vi "CameraVision.vi"(8 "error in (no error)":errorcluster, 9 "Com-in":refnum<queue>, 10 "Com-out":refnum<queue>) -> (0 "error out":errorcluster)   [LabVIEW 2013, in "CameraVision.lvlib"]
doc: "This vi is the main component of the CameraVision software.\n\nThe software is made for the acquisition, processing and storage of images. Specifically using one or two CMOS cameras and a SiliconSoftware framegrabber. The cameras can be any type compatible with the framegrabber, though the software is only tested with PhotonFocus CMOS-cameras of the MV-D1312-240-CL model. In this case a separate software called 'PFRemote', provided by PhotonFocus, is necessary for changing camera parameters.\n\nThe main program controls are on the top of the window. User-configurable settings are grouped per category on the left panel. All outputs are displayed at the right side of the window. Different display configurations can be chosen using the tabs."
uses:
  CameraVision.lvlib
  Sources/UI/Settings-source.ctl
  Sources/UI/Camera-selector.ctl
  Sources/UI/Image-selector.ctl
  Sources/Main/Configuration/Configuration-parameters-gui.ctl
  Sources/Main/Storage/Storage-parameters-gui.ctl
  Sources/Main/Storage/Storage-types.ctl
  Sources/Main/Acquisition/Acquisition-parameters-gui.ctl
  Sources/Main/Acquisition/Trigger-modes.ctl
  Sources/Main/Acquisition/Exposure-modes.ctl
  Sources/Main/Analysis/Characteristics-cluster.ctl
  Sources/Main/Correction/Correction-parameters-gui.ctl
  Sources/Main/Correction/Smoothing.ctl
  Sources/Main/Correction/Background-correction.ctl
  Sources/Main/Analysis/Analysis-parameters-gui.ctl
  Sources/Main/Temperature/Temperature-parameters-gui.ctl
  Sources/Main/Mapping/Mapping-parameters-gui.ctl
  Sources/Main/Mapping/Mapping-characteristic.ctl
  Sources/Main/Temperature/Temperature-characteristics.ctl
  SA-SLMAPI/Sources/Message.lvclass
  Sources/UI/Status-overview.ctl
  Sources/UI/Module-states.ctl
  Sources/Main/Filter/Filter-parameters-gui.ctl
  Sources/Main/Filter/Filter-settings.ctl
  Sources/Main/Filter/Filter-characteristic.ctl
  Sources/Main/Filter/Filter-apply.ctl
  Sources/Main/Main-actions.ctl
  Sources/Main/Application-states.ctl
  Sources/Main/CV-Main.lvclass
  Sources/UI/CV-UI.lvclass
  Sources/Main/Configuration/CV-Configuration.lvclass
  Sources/Main/Storage/CV-Storage.lvclass
  Sources/Main/Acquisition/CV-Acquisition.lvclass
  Sources/Main/Analysis/CV-Analysis.lvclass
  Sources/Main/Correction/CV-Correction.lvclass
  Sources/Main/Temperature/CV-Temperature.lvclass
  Sources/Main/Mapping/CV-Mapping.lvclass
  Sources/Main/Filter/CV-Filter.lvclass
panel:
  in  "Start acquisition":bool
  in  "Manual trigger":bool
  in  "Camera selector":T1 caption="Display camera"
  in  "Image type selector":T2 caption="Display image"
  in  "Batch browser":i32(slide) caption="Browse batch" min=-29 max=0 step=1
  in  "Image refresh":bool
  in  "Import images":bool
  in  "Save settings":bool
  in  "Load settings":bool
  in  "Settings type":T3
  in  "Stop acquisition":bool
  in  "Activate":bool
  in  "Show info":bool
  in  "Parameter tabs":T4(tab) caption="Parameters"
  in  "Configuration params":T5={"Number of cameras"=1, "Camera 1 port"=enum."A", "ROI width"=1248, "ROI height"=1082, "Reset ROI"=FALSE, "Width scale"=0.05, "Height scale"=0.05, "Center Y cam. 1"=541, "Center X cam. 1"=624, "Center Y cam. 2"=541, "Center X cam. 2"=624} {"Center X cam. 2" min=4 max=1244 step=8; "Center Y cam. 2" min=1 max=1082 step=1; "Center X cam. 1" min=4 max=1244 step=8; "Center Y cam. 1" min=1 max=1082 step=1; "Height scale" min=0.001 step=0.001 format="%.3f"; "Width scale" min=0.001 step=0.001 format="%.3f"; "Number of cameras" min=1 max=2 step=1; "ROI width" min=8 max=1248 step=8; "ROI height" min=1 max=1082 step=1}
  in  "Acquisition params":T6={"Acquisition mode"=enum."Continuous", "Batch size"=0, "Image buffer size"=0, "Trigger mode"=enum."Camera timed (not sync.)", "Duration HH"=1.0, "Acquisition start"=enum."Immediate", "Duration SS"=0.0, "Duration MM"=0.0, "Start time"=timestamp(0 s since 1904-01-01), "Max. frame rate"=5.0, "Exposure time cam. 1"=1.0, "Exposure time cam. 2"=1.0, "Exposure mode"=enum."Linear", "Value 1"=17.0, "Value 2"=14.0, "Time 1"=1000.0, "Time 2"=1000.0} {"Exposure time cam. 2" min=0.01 step=0.01 format="%#.2g"; "Exposure time cam. 1" min=0.01 step=0.01 format="%#.2g"; "Max. frame rate" min=0.0001 max=1000000.0 format="%#.4g"; "Start time" format="%<%X\n%x>T"; "Duration MM" min=0 max=59 step=1 format="%02.0f"; "Duration SS" min=0 max=59 step=1 format="%02.0f"; "Duration HH" min=0 step=1 format="%02.0f"; "Image buffer size" min=1 max=10000 step=1 format="%#.0f"; "Batch size" min=1 max=50000 step=1}
  in  "Processing selector":u32(ring) items=["Correction", "Analysis", "Temperature", "Mapping"]
  in  "Processing tabs":T9(tab)
  in  "Correction params":T10={"Background correction"=FALSE, "Hot-pixel correction"=FALSE, "Black image cam. 1"=path "C:/CameraVision/Black images/Black-CameraA-Full.bmp", "Black image cam. 2"=path "C:/CameraVision/Black images/Black-CameraB-Full.bmp", "Y-shift"=0, "X-shift"=0, "Correlation algorithm"=enum."Fixed shift", "Noise treshold"=25.0, "Smoothing algorithm"=enum."Noise tresholding", "2nd image correlation"=FALSE, "Image smoothing"=FALSE, "Background correction method"=enum."Hardware"} {"Noise treshold" min=0 max=255 step=1}
  in  "Analysis params":T13={"Binarization treshold"=150.0, "Image characteristics"=FALSE, "Melt-pool characteristics"=FALSE} {"Binarization treshold" min=0 max=255 step=1}
  in  "Temperature params":T14={"Temperature field"=FALSE, "Ratio correction factor"=1.0, "Temperature value"=FALSE, "Y-coord."=0.0, "X-coord."=0.0, "Averaging center"=enum."Melt-pool center", "Averaging shape"=enum."Point", "Minor axis"=0.0, "Major axis"=0.0} {"Major axis" min=0.0; "Minor axis" min=0.0; "Ratio correction factor" min=0.0 step=0.0001 format="%#.4g"}
  in  "Mapping params":T15 {"Jump speed" min=1; "Default mark speed" min=1; "Start off-set" step=0.0001}
  in  "Storage params":T17={"Base file name"="Test", "Storage directory"=path "C:/CameraVision/Results", "Save what?"={"Original"=FALSE, "Corrected"=FALSE, "Binary"=FALSE, "Temperature"=FALSE, "Characteristics"=FALSE, "Mapping"=FALSE, "TemperatureValues"=FALSE}, "Image file type"=enum."PNG", "Comments"="", "Storage mode"=enum."1 file for all layers ", "Start iteration/layer"=0}
  in  "Filter params":T19
  out "Storage buffer":dbl(slide) scale=0.0..1.0
  out "Framerate":dbl caption="Frame rate [fps]" format="%06.1f"
  out "Status overview":T23
  out "Frametime":dbl caption="Process time [ms/frame]" format="%04.0g"
  out "Process buffer":dbl(slide) scale=0.0..1.0
  out "Total disk space":dbl caption="Total [GB]" format="%05.1f"
  out "Free disk space":dbl caption="Free [GB]    /" format="%05.1f"
  out "Current image":i32 caption="Current image #" format="%06.0f"
  in  "Displays":T25(tab)=enum."Dual view"
  out "Browser":T26(plugin-control)
  out "Camera 2":T26(plugin-control)
  out "Camera 1":T26(plugin-control)
  out "Temper characteristics":T27 caption="Temperature" {"Stand. dev. temperature" format="%#.1f"; "Min. temperature" format="%#.0f"; "Max. temperature" format="%#.0f"; "Average temperature" format="%#.0f"}
  out "Characteristics":T28 caption="Image/melt-pool"
  out "Histogram":T29(graph)
  out "Information":T26(plugin-control)
  out "Camera 2 chart":dbl[][](graph) caption="Camera 2 - characteristics chart"
  out "Camera 1 chart":dbl[][](graph) caption="Camera 1 - characteristics chart"
  out "Temperature":dbl[][](graph) caption="Temperature [°C]"
  out "Map":dbl[][](graph)
  in  "Map characteristic":T16
  out "State":string caption="Status:"
  out "Action":string caption="Action:"
  # ":"
  # ":"
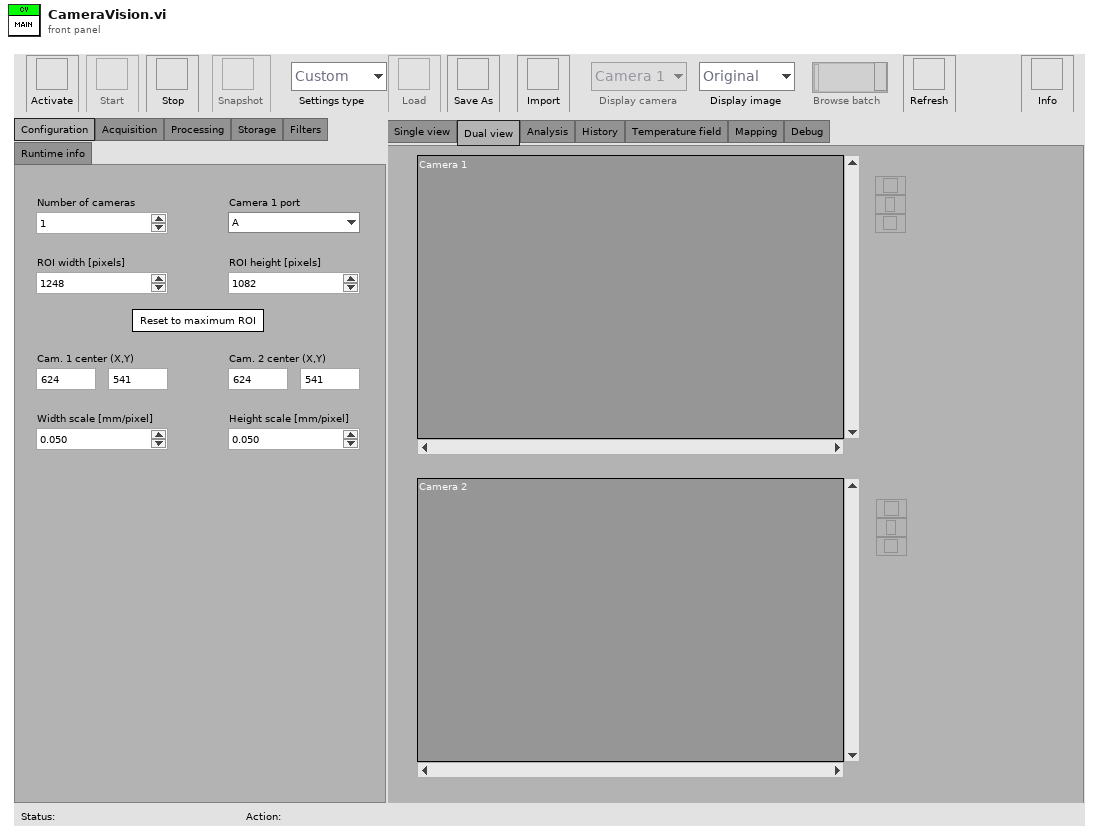
[diagram p1: front panel]
types:
  T1 = typedef "CameraVision.lvlib/CV-UI.lvclass/Camera-selector.ctl" = enum16{"Camera 1", "Camera 2"}
  T2 = typedef "CameraVision.lvlib/CV-UI.lvclass/Image-selector.ctl" = enum16{"Original", "Corrected", "Binary"}
  T3 = typedef "CameraVision.lvlib/CV-UI.lvclass/Settings-source.ctl" = enum16{"Custom", "Default", "Last used", "File"}
  T4 = enum32{"Configuration", "Acquisition", "Processing", "Storage", "Filters", "Runtime info"}
  T5 = typedef "CameraVision.lvlib/CV-Configuration.lvclass/Configuration-parameters-gui.ctl" = cluster{"Number of cameras":i32, "Camera 1 port":enum16{"A", "B"}, "ROI width":u32, "ROI height":u32, "Reset ROI":bool, "Width scale":dbl, "Height scale":dbl, "Center Y cam. 1":i32, "Center X cam. 1":i32, "Center Y cam. 2":i32, "Center X cam. 2":i32}
  T6 = typedef "CameraVision.lvlib/CV-Acquisition.lvclass/Acquisition-parameters-gui.ctl" = cluster{"Acquisition mode":enum16{"Continuous", "Continuous batch", "Single batch", "Single batch -delayed"}, "Batch size":i32, "Image buffer size":i32, "Trigger mode":T7, "Duration HH":sgl, "Acquisition start":enum16{"Immediate", "Post-phoned"}, "Duration SS":sgl, "Duration MM":sgl, "Start time":timestamp, "Max. frame rate":dbl, "Exposure time cam. 1":dbl, "Exposure time cam. 2":dbl, "Exposure mode":T8, "Value 1":dbl, "Value 2":dbl, "Time 1":dbl, "Time 2":dbl}
  T7 = typedef "CameraVision.lvlib/CV-Acquisition.lvclass/Trigger-modes.ctl" = enum16{"Camera timed (not sync.)", "Framegrabber timed (sync.)", "Software timed (sync.)", "External timing (sync.)", "Manual (sync.)", "Gated - camera (not sync.)", "Gated - grabber (sync.)", "Gated - software (sync.)", "Gated - external (sync.)"}
  T8 = typedef "CameraVision.lvlib/CV-Acquisition.lvclass/Exposure-modes.ctl" = enum16{"Linear", "LinLog"}
  T9 = enum32{"Correction", "Analysis", "Temperature", "Mapping"}
  T10 = typedef "CameraVision.lvlib/CV-Correction.lvclass/Correction-parameters-gui.ctl" = cluster{"Background correction":bool, "Hot-pixel correction":bool, "Black image cam. 1":path, "Black image cam. 2":path, "Y-shift":i32, "X-shift":i32, "Correlation algorithm":enum16{"Fixed shift", "Cross-correlation", "Cross-correlation (5steps)", "Melt-pool center"}, "Noise treshold":sgl, "Smoothing algorithm":T11, "2nd image correlation":bool, "Image smoothing":bool, "Background correction method":T12}
  T11 = typedef "CameraVision.lvlib/CV-Correction.lvclass/Smoothing.ctl" = enum16{"Noise tresholding", "NT+Median filter", "NT+Gaussian filter"}
  T12 = typedef "CameraVision.lvlib/CV-Correction.lvclass/Background-correction.ctl" = enum16{"Hardware", "Software"}
  T13 = typedef "CameraVision.lvlib/CV-Analysis.lvclass/Analysis-parameters-gui.ctl" = cluster{"Binarization treshold":sgl, "Image characteristics":bool, "Melt-pool characteristics":bool}
  T14 = typedef "CameraVision.lvlib/CV-Temperature.lvclass/Temperature-parameters-gui.ctl" = cluster{"Temperature field":bool, "Ratio correction factor":dbl, "Temperature value":bool, "Y-coord.":dbl, "X-coord.":dbl, "Averaging center":enum16{"Fixed coordinates (pixel)", "Fixed coordinates (mm)", "Melt-pool center"}, "Averaging shape":enum16{"Point", "Circle", "Ellipse"}, "Minor axis":dbl, "Major axis":dbl}
  T15 = typedef "CameraVision.lvlib/CV-Mapping.lvclass/Mapping-parameters-gui.ctl" = cluster{"Enable mapping":bool, "Automatic timing":bool, "Scan pattern file":path, "Start off-set":dbl, "Default map characteristic":T16, "Default mark speed":i32, "Jump speed":i32}
  T16 = typedef "CameraVision.lvlib/CV-Mapping.lvclass/Mapping-characteristic.ctl" = enum16{"Average intensity [0-255]", "Peak intensity [0-255]", "Melt-pool size [mm²]", "Melt-pool aspect ratio []", "Melt-pool fragments []", "Average temperature [°C]", "Max. temperature [°C]", "Min. temperature [°C]", "Std. dev. temperature [°C]"}
  T17 = typedef "CameraVision.lvlib/CV-Storage.lvclass/Storage-parameters-gui.ctl" = cluster{"Base file name":string, "Storage directory":path, "Save what?":T18, "Image file type":enum16{"JPG", "BMP", "PNG"}, "Comments":string, "Storage mode":enum16{"1 file per layer", "1 file for all layers "}, "Start iteration/layer":u16}
  T18 = typedef "CameraVision.lvlib/CV-Storage.lvclass/Storage-types.ctl" = cluster{"Original":bool, "Corrected":bool, "Binary":bool, "Temperature":bool, "Characteristics":bool, "Mapping":bool, "TemperatureValues":bool}
  T19 = typedef "CameraVision.lvlib/CV-Filter.lvclass/Filter-parameters-gui.ctl" = cluster{"Filter array":T20[], "Storage filters":T22}
  T20 = typedef "CameraVision.lvlib/CV-Filter.lvclass/Filter-settings.ctl" = cluster{"Characteristic":T21, "Monitor":bool, "Min.":dbl, "Max.":dbl, "Min. Thres.":dbl, "Min. Dur.":u16, "Report":bool}
  T21 = typedef "CameraVision.lvlib/CV-Filter.lvclass/Filter-characteristic.ctl" = enum16{"Average intensity [0-255]", "Peak intensity [0-255]", "Melt-pool size [mm²]", "Melt-pool aspect ratio []", "Melt-pool fragments []", "Melt-pool position X [pixel]", "Melt-pool position Y [pixel]", "Average temperature [°C]", "Max. temperature [°C]", "Min. temperature [°C]", "Std. dev. temperature [°C]"}
  T22 = typedef "CameraVision.lvlib/CV-Filter.lvclass/Filter-apply.ctl" = cluster{"Filter images":bool, "Filter characteristics":bool, "Filter temperature":bool}
  T23 = typedef "CameraVision.lvlib/CV-UI.lvclass/Status-overview.ctl" = cluster{"Camera hardware":T24, "Framegrabber":T24, "External timing":T24, "Image acquisition":T24, "Image processing ":T24, "Temperature":T24, "Map":T24, "Storage filter":T24, "Image storage":T24, "Charact. storage":T24, "Temperature storage":T24, "Camera hardware G":bool, "Camera hardware R":bool, "Framegrabber G":bool, "Framegrabber R":bool, "External timing G":bool, "External timing R":bool, "Image acquisition G":bool, "Image acquisition R":bool, "Image processing G":bool, "Image processing R":bool, "Temperature G":bool, "Temperature R":bool, "Map G":bool, "Map R":bool, "Storage filter G":bool, "Storage filter R":bool, "Image storage G":bool, "Image storage R":bool, "Charact storage G":bool, "Charact storage R":bool, "Temperature storage G":bool, "Temperature storage R":bool}
  T24 = typedef "CameraVision.lvlib/CV-UI.lvclass/Module-states.ctl" = enum16{"Inactive", "Active", "Data-loss", "Error", "Simulation", "Synchronizing", "Initialized", "Released"}
  T25 = enum32{"Single view", "Dual view", "Analysis", "History", "Temperature field", "Mapping", "Debug"}
  T26 = typedef "IMAQ Image.ctl" = refnum<image>
  T27 = typedef "CameraVision.lvlib/CV-Temperature.lvclass/Temperature-characteristics.ctl" = cluster{"Average temperature ":dbl, "Max. temperature":dbl, "Min. temperature":dbl, "Stand. dev. temperature":dbl, "Datapoints":dbl}
  T28 = typedef "CameraVision.lvlib/CV-Analysis.lvclass/Characteristics-cluster.ctl" = cluster{"Average intensity":dbl, "Peak intensity":dbl, "Melt-pool size":dbl, "Melt-pool aspect ratio":dbl, "Melt-pool fragments":dbl, "Centre of mass X":dbl, "Centre of mass Y":dbl, "Orientation":dbl}
  T29 = cluster{"Starting Value":sgl, "Incremental Value":sgl, "Histogram":u32[]}
  T30 = typedef "CameraVision.lvlib/CV-Main.lvclass/Main-actions.ctl" = enum16{"Idle", "Initialize", "Load defaults", "Update settings", "Check settings", "Save settings", "Save settings with dialog", "Load settings", "Load data", "Activate", "Start", "Wait for start signal", "Acquire & process", "Iterate", "Stop", "Refresh display", "Refresh status", "View camera settings", "View grabber settings", "Exit"}
  T31 = typedef "CameraVision.lvlib/CV-Main.lvclass/Application-states.ctl" = enum16{"Idle", "Initialized", "Configured", "Activated", "Started", "Stopped", "Reset", "Error", "Exited"}
  T32 = enum16{"Continuous", "Continuous batch", "Single batch", "Single batch -delayed"}
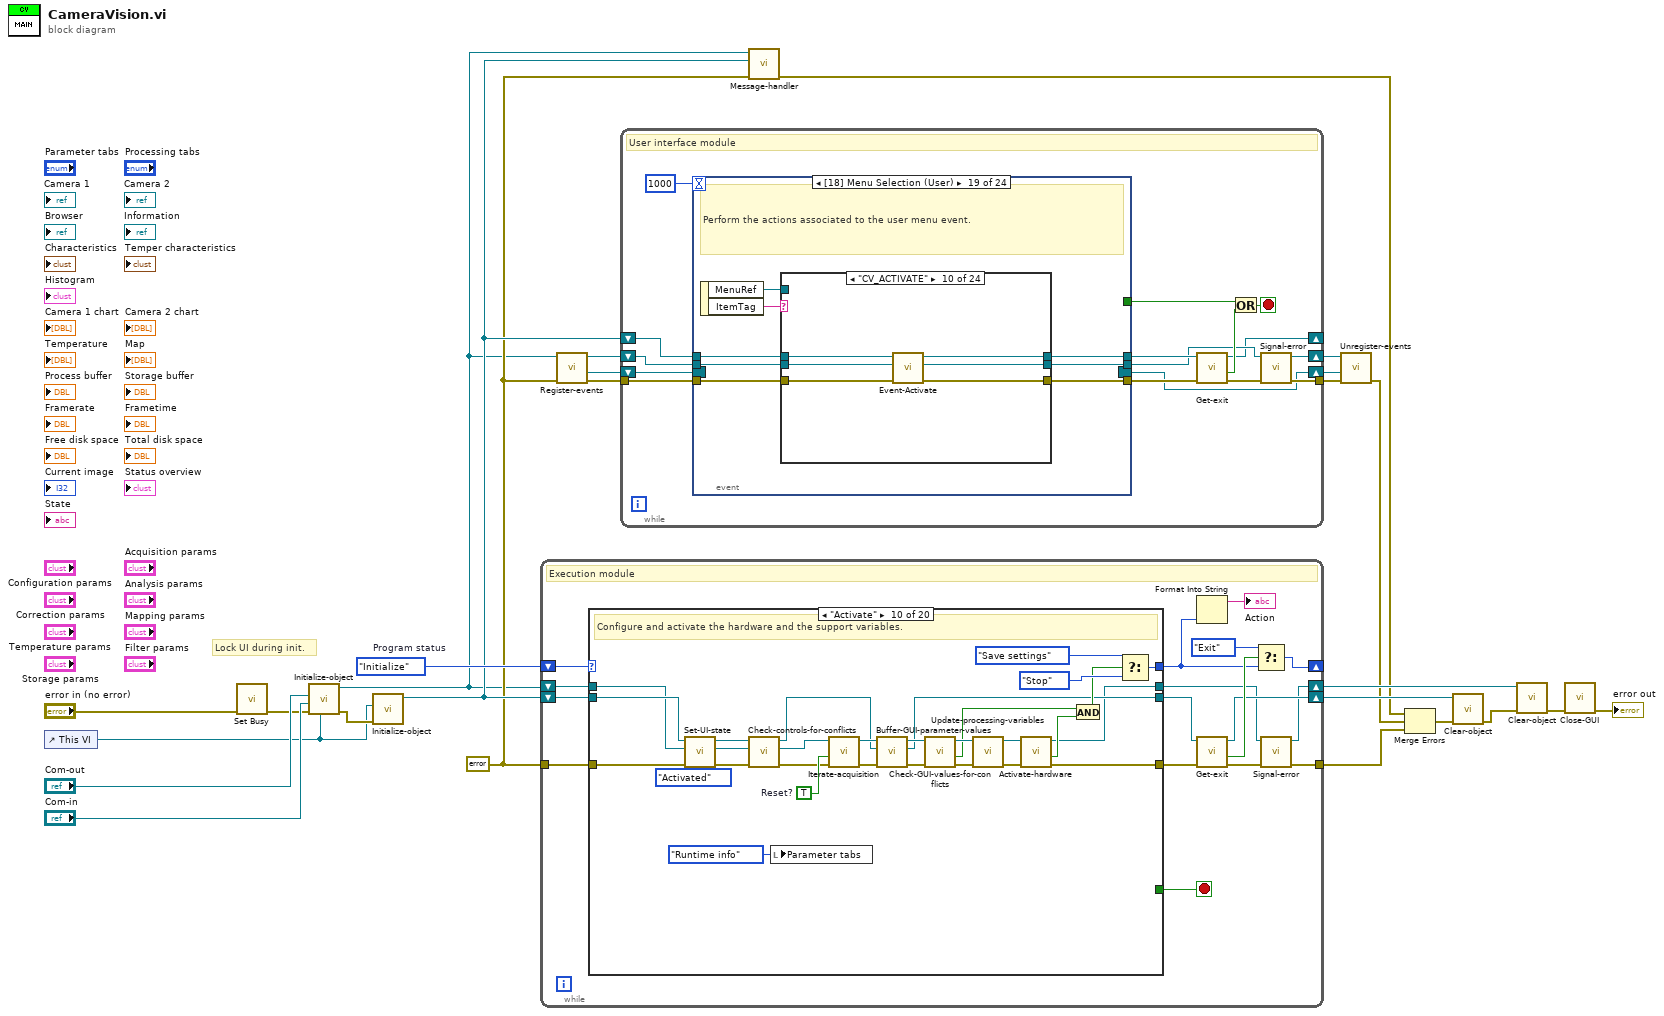
[diagram p0: block diagram]
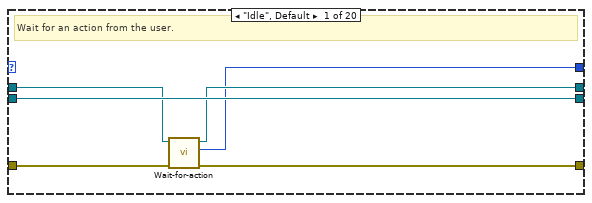
[diagram p2: hidden frame]
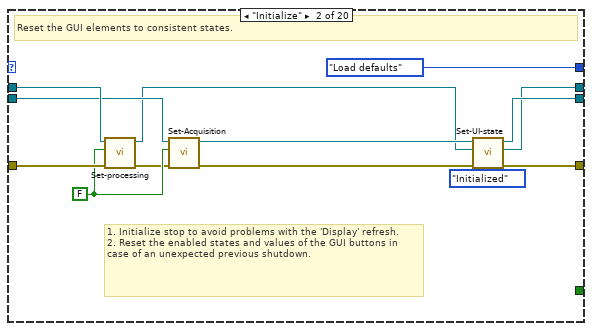
[diagram p3: hidden frame]
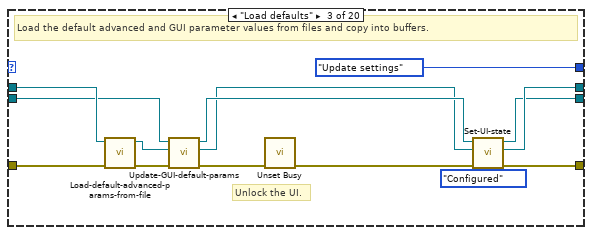
[diagram p4: hidden frame]
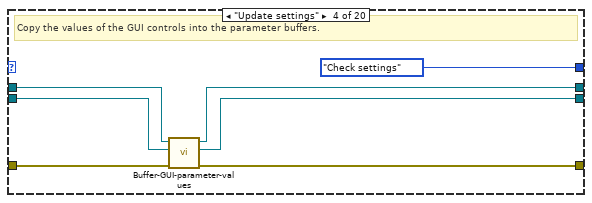
[diagram p5: hidden frame]
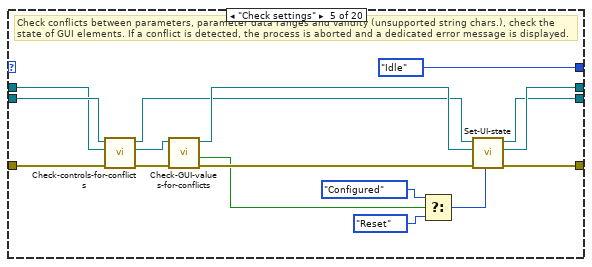
[diagram p6: hidden frame]
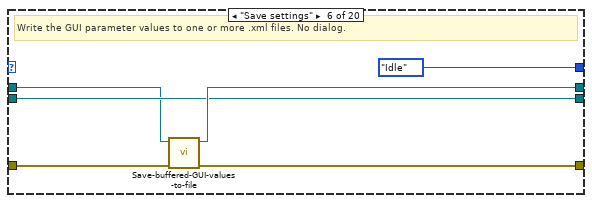
[diagram p7: hidden frame]
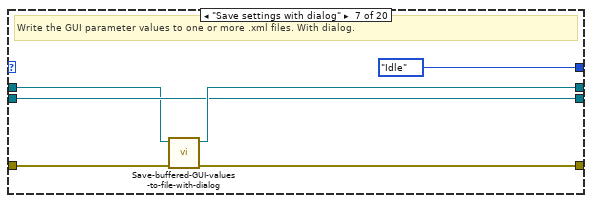
[diagram p8: hidden frame]
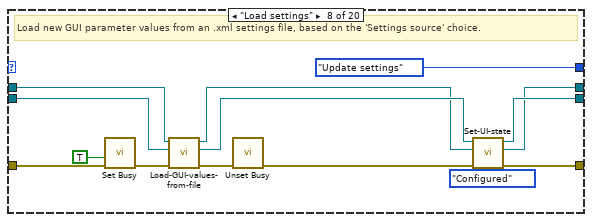
[diagram p9: hidden frame]
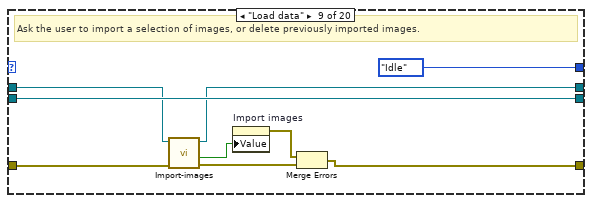
[diagram p10: hidden frame]
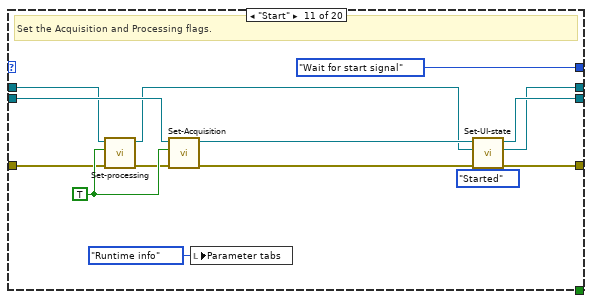
[diagram p11: hidden frame]
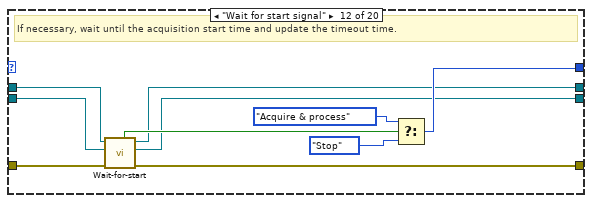
[diagram p12: hidden frame]
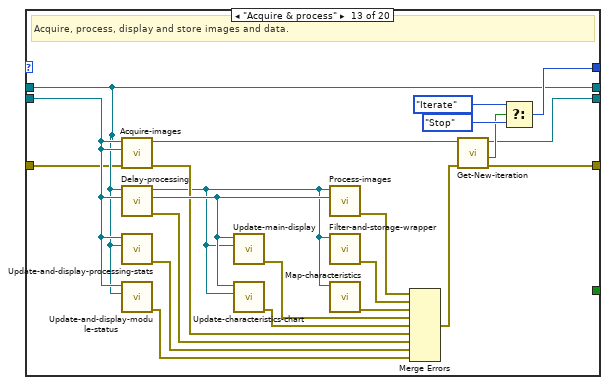
[diagram p13: hidden frame]
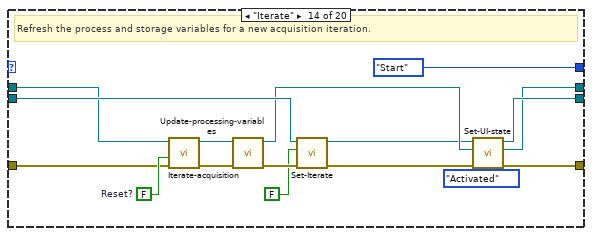
[diagram p14: hidden frame]
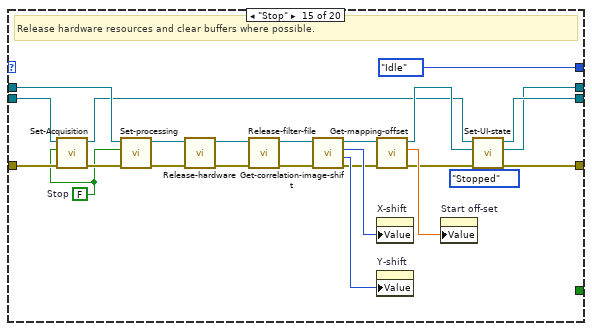
[diagram p15: hidden frame]
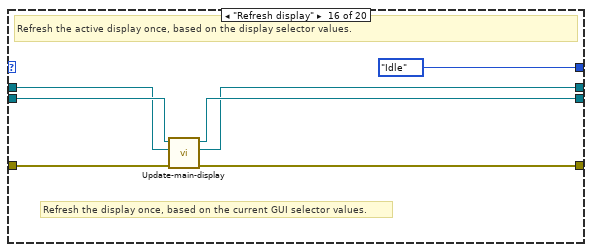
[diagram p16: hidden frame]
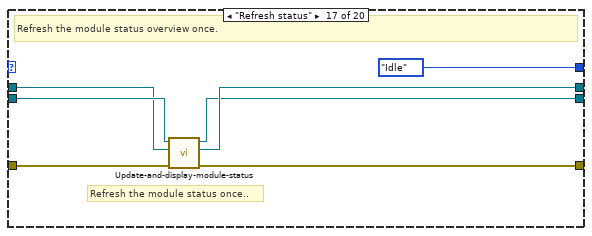
[diagram p17: hidden frame]
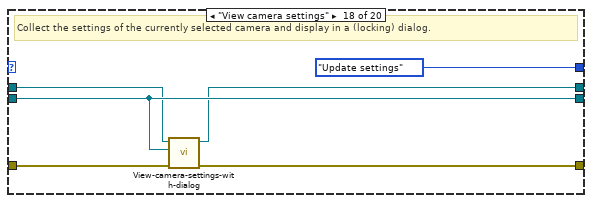
[diagram p18: hidden frame]
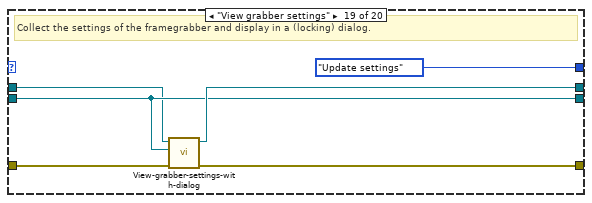
[diagram p19: hidden frame]
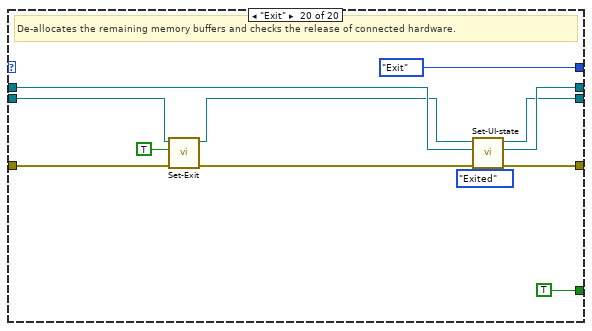
[diagram p20: hidden frame]
diagram:
  w8 = errorcluster {"status"=FALSE, "code"=0, "source"=""} ("error constant")
  w25 = Main-actions."Initialize"  # Program status
  # "Lock UI during init."
  n1 = control-ref of="This VI"() -> (w14:refnum<vi>)
  n2 = call <vilib>:"Set Busy.vi"("error in (no error)"="error in (no error)") -> ("error out"=w1:errorcluster)  [unwired: 9 in, 1 out]
  n3 = call "Initialize-object.vi"("Main VI ref"=w14, "error in (no error)"=w1, "Com-in"="Com-in", "Com-out"="Com-out") -> ("error out"=w21:errorcluster, "Data ref."=w7:refnum<data-value>)  [unwired: 6 in]
  n4 = call "Initialize-object.vi"("error in"=w21, "Main VI ref"=w14) -> ("UI ref."=w15:refnum<data-value>)  [unwired: 8 in, 1 out]
  n5 = while {
    shift-right: [w34] -> _
    shift-left: w25 -> [w39]
    shift-right: [w30] -> w20
    shift-left: w15 -> [w38]
    shift-right: [w27] -> w22
    shift-left: w7 -> [w37]
    tunnel: w8 -> [w41]
    tunnel: [w28] -> w18
    stop <- w42 stop-if-true
    # "Execution module"
    n6 = case shown="\"Activate\"" w39 {
      tunnel: w41 -> [w47 w57 w74 w82 w96 w101 w107 w124 w133 w142 w166 w186 w196 w210 w227 w254 w255 w262 w268 w282]
      tunnel: [w43 w59 w65 w81 w92 w102 w108 w116 w125 w134 w172 w177 w201 w217 w237 w252 w256 w264 w271 w276] -> w36
      tunnel: [w44 Main-actions."Load defaults" ("MainStateSelector") Main-actions."Update settings" ("MainStateSelector") Main-actions."Check settings" ("MainStateSelector") Main-actions."Idle" ("MainStateSelector") Main-actions."Idle" ("MainStateSelector") Main-actions."Idle" ("MainStateSelector") Main-actions."Update settings" ("MainStateSelector") Main-actions."Idle" ("MainStateSelector") w160 Main-actions."Wait for start signal" ("MainStateSelector") w183 w206 Main-actions."Start" ("MainStateSelector") Main-actions."Idle" ("MainStateSelector") Main-actions."Idle" ("MainStateSelector") Main-actions."Idle" ("MainStateSelector") Main-actions."Update settings" ("MainStateSelector") Main-actions."Update settings" ("MainStateSelector") Main-actions."Exit" ("MainStateSelector")] -> w31
      tunnel: [_ _ _ _ _ _ _ _ _ _ _ _ _ _ _ _ _ _ _ TRUE] -> w42
      tunnel: w38 -> [w48 w56 w72 w78 w97 w103 w109 w114 w131 w140 w175 w180 w198 w219 w229 w251 w260 w266 w270 w283]
      tunnel: [w48 w58 w68 w77 w88 w103 w109 w120 w131 w136 w171 w178 w199 w218 w238 w250 w257 w266 w270 w277] -> w35
      tunnel: w37 -> [w46 w60 w73 w79 w95 w100 w106 w113 w130 w138 w167 w181 w197 w211 w241 w248 w259 w263 w269 w279]
      tunnel: [w45 w52 w70 w76 w91 w104 w110 w119 w129 w135 w170 w179 w197 w214 w231 w249 w258 w265 w272 w280] -> w26
      frame "Idle", Default {
        # "Wait for an action from the user."
        n7 = call "Wait-for-action.vi"("error in (no error)"=w47, "Data ref. in"=w46) -> ("error out"=w43:errorcluster, "Next action"=w44:T30, "Data ref."=w45:refnum<data-value>)  [unwired: 7 in]
      }
      frame "Initialize" {
        w54 = FALSE ("Stop")
        # "1. Initialize stop to avoid problems with the 'Display' refresh.\n2. Reset the enabled states and values of the GUI buttons in case of an unexpected previous shutdown."
        # "Reset the GUI elements to consistent states."
        n8 = call "Set-processing.vi"("error in (no error)"=w57, "Processing"=w54, "Data ref. in"=w60) -> ("error out"=w51:errorcluster, "Data ref."=w53:refnum<data-value>)  [unwired: 7 in]
        n9 = call "Set-Acquisition.vi"("error in (no error)"=w51, "Acquisition"=w54, "UI ref. in"=w56) -> ("error out"=w50:errorcluster, "UI ref."=w55:refnum<data-value>)  [unwired: 7 in]
        n10 = call "Set-UI-state.vi"("State"=Application-states."Initialized", "error in"=w50, "Data ref. in"=w53, "UI ref. in"=w55) -> ("error IO"=w59:errorcluster, "Data ref."=w52:refnum<data-value>, "UI ref."=w58:refnum<data-value>)  [unwired: 5 in]
      }
      frame "Load defaults" {
        # "Unlock the UI."
        # "Load the default advanced and GUI parameter values from files and copy into buffers."
        n11 = call "Load-default-advanced-params-from-file.vi"("error in"=w74, "Data ref. in"=w73) -> ("error IO"=w71:errorcluster, "Data ref."=w64:refnum<data-value>)  [unwired: 8 in]
        n12 = call "Update-GUI-default-params.vi"("error in"=w71, "Data ref. in"=w64, "UI ref. in"=w72) -> ("error IO"=w66:errorcluster, "Data ref."=w63:refnum<data-value>, "UI ref."=w69:refnum<data-value>)  [unwired: 6 in]
        n13 = call <vilib>:"Unset Busy.vi"("error in (no error)"=w66) -> ("error out"=w67:errorcluster)  [unwired: 10 in]
        n14 = call "Set-UI-state.vi"("State"=Application-states."Configured", "error in"=w67, "Data ref. in"=w63, "UI ref. in"=w69) -> ("error IO"=w65:errorcluster, "Data ref."=w70:refnum<data-value>, "UI ref."=w68:refnum<data-value>)  [unwired: 5 in]
      }
      frame "Update settings" {
        # "Copy the values of the GUI controls into the parameter buffers."
        n15 = call "Buffer-GUI-parameter-values.vi"("error in"=w82, "UI ref. in"=w78, "Data ref. in"=w79) -> ("error IO"=w81:errorcluster, "UI ref."=w77:refnum<data-value>, "Data ref."=w76:refnum<data-value>)  [unwired: 6 in]
      }
      frame "Check settings" {
        # "Check conflicts between parameters, parameter data ranges and validity (unsupported string chars.), check the state of GUI elements. If a conflict is detected, the process is aborted and a dedicated error message is displayed."
        n16 = call "Check-controls-for-conflicts.vi"("error in (no error)"=w96, "Data ref. in"=w95, "UI ref. in"=w97) -> ("error out"=w93:errorcluster, "Data ref."=w94:refnum<data-value>, "UI ref."=w89:refnum<data-value>)  [unwired: 6 in]
        n17 = call "Check-GUI-values-for-conflicts.vi"("error in (no error)"=w93, "Data ref. in"=w94) -> ("error out"=w87:errorcluster, "Passed?"=w84:bool, "Data ref."=w90:refnum<data-value>)  [unwired: 7 in]
        n18 = Select(t=Application-states."Configured" ("State"), s=w84, f=Application-states."Reset" ("State")) -> (s? t:f=w83:T31)
        n19 = call "Set-UI-state.vi"("State"=w83, "error in"=w87, "Data ref. in"=w90, "UI ref. in"=w89) -> ("error IO"=w92:errorcluster, "Data ref."=w91:refnum<data-value>, "UI ref."=w88:refnum<data-value>)  [unwired: 5 in]
      }
      frame "Save settings" {
        # "Write the GUI parameter values to one or more .xml files. No dialog."
        n20 = call "Save-buffered-GUI-values-to-file.vi"("error in"=w101, "Data ref. in"=w100) -> ("error IO"=w102:errorcluster, "Data ref."=w104:refnum<data-value>)  [unwired: 8 in]
      }
      frame "Save settings with dialog" {
        # "Write the GUI parameter values to one or more .xml files. With dialog."
        n21 = call "Save-buffered-GUI-values-to-file-with-dialog.vi"("error in"=w107, "Data ref. in"=w106) -> ("error IO"=w108:errorcluster, "Data ref."=w110:refnum<data-value>)  [unwired: 8 in]
      }
      frame "Load settings" {
        # "Load new GUI parameter values from an .xml settings file, based on the 'Settings source' choice."
        n22 = call <vilib>:"Set Busy.vi"("error in (no error)"=w124, "disable click? (T)"=TRUE) -> ("error out"=w123:errorcluster)  [unwired: 8 in, 1 out]
        n23 = call "Load-GUI-values-from-file.vi"("error in"=w123, "UI ref. in"=w114, "Data ref. in"=w113) -> ("error IO"=w118:errorcluster, "UI ref."=w115:refnum<data-value>, "Data ref."=w112:refnum<data-value>)  [unwired: 6 in]
        n24 = call <vilib>:"Unset Busy.vi"("error in (no error)"=w118) -> ("error out"=w117:errorcluster)  [unwired: 10 in]
        n25 = call "Set-UI-state.vi"("State"=Application-states."Configured", "error in"=w117, "Data ref. in"=w112, "UI ref. in"=w115) -> ("error IO"=w116:errorcluster, "Data ref."=w119:refnum<data-value>, "UI ref."=w120:refnum<data-value>)  [unwired: 5 in]
      }
      frame "Load data" {
        # "Ask the user to import a selection of images, or delete previously imported images."
        n26 = call "Import-images.vi"("error in"=w133, "Data ref. in"=w130) -> ("error IO"=w127:errorcluster, "Imported?"=w128:bool, "Data ref."=w129:refnum<data-value>)  [unwired: 7 in]
        n27 = property on="Import images" class="Bool (strict)"("Value"=w128) -> (error out=w126:errorcluster)  [unwired: 2 in, 1 out]
        n28 = Merge Errors(w126, w127) -> (w125:errorcluster)
      }
      frame "Activate" {
        w159 = TRUE  # Reset?
        # "Configure and activate the hardware and the support variables."
        n29 = call "Set-UI-state.vi"("State"=Application-states."Activated", "error in"=w142, "Data ref. in"=w138, "UI ref. in"=w140) -> ("error IO"=w141:errorcluster, "Data ref."=w137:refnum<data-value>, "UI ref."=w139:refnum<data-value>)  [unwired: 5 in]
        n30 = call "Check-controls-for-conflicts.vi"("error in (no error)"=w141, "Data ref. in"=w137, "UI ref. in"=w139) -> ("error out"=w151:errorcluster, "Data ref."=w152:refnum<data-value>, "UI ref."=w149:refnum<data-value>)  [unwired: 6 in]
        n31 = local write "Parameter tabs"(T4."Runtime info" ("Parameters")) -> ()
        n32 = call "Iterate-acquisition.vi"("error in"=w151, "Reset?"=w159, "Data ref. in"=w152) -> ("error IO"=w154:errorcluster, "Data ref."=w155:refnum<data-value>)  [unwired: 7 in]
        n33 = call "Buffer-GUI-parameter-values.vi"("error in"=w154, "UI ref. in"=w149, "Data ref. in"=w155) -> ("error IO"=w148:errorcluster, "UI ref."=w136:refnum<data-value>, "Data ref."=w150:refnum<data-value>)  [unwired: 6 in]
        n34 = call "Check-GUI-values-for-conflicts.vi"("error in (no error)"=w148, "Data ref. in"=w150) -> ("error out"=w147:errorcluster, "Passed?"=w144:bool, "Data ref."=w153:refnum<data-value>)  [unwired: 7 in]
        n35 = call "Update-processing-variables.vi"("error in (no error)"=w147, "Data ref. in"=w153) -> ("error out"=w157:errorcluster, "Data ref."=w158:refnum<data-value>)  [unwired: 8 in]
        n36 = call "Activate-hardware.vi"("error in (no error)"=w157, "Data ref. in"=w158) -> ("error out"=w134:errorcluster, "Succes?"=w145:bool, "Data ref."=w135:refnum<data-value>)  [unwired: 7 in]
        n37 = And(x=w144, y=w145) -> (x .and. y?=w146:bool)
        n38 = Select(t=Main-actions."Save settings" ("MainStateSelector"), s=w146, f=Main-actions."Stop" ("MainStateSelector")) -> (s? t:f=w160:T30)
      }
      frame "Start" {
        w169 = TRUE ("Stop")
        # "Set the Acquisition and Processing flags."
        n39 = call "Set-processing.vi"("error in (no error)"=w166, "Processing"=w169, "Data ref. in"=w167) -> ("error out"=w165:errorcluster, "Data ref."=w168:refnum<data-value>)  [unwired: 7 in]
        n40 = call "Set-Acquisition.vi"("error in (no error)"=w165, "Acquisition"=w169, "UI ref. in"=w175) -> ("error out"=w173:errorcluster, "UI ref."=w174:refnum<data-value>)  [unwired: 7 in]
        n41 = local write "Parameter tabs"(T4."Runtime info" ("Parameters")) -> ()
        n42 = call "Set-UI-state.vi"("State"=Application-states."Started", "error in"=w173, "Data ref. in"=w168, "UI ref. in"=w174) -> ("error IO"=w172:errorcluster, "Data ref."=w170:refnum<data-value>, "UI ref."=w171:refnum<data-value>)  [unwired: 5 in]
      }
      frame "Wait for start signal" {
        # "If necessary, wait until the acquisition start time and update the timeout time."
        n43 = call "Wait-for-start.vi"("error in"=w186, "UI ref. in"=w180, "Data ref. in"=w181) -> ("error IO"=w177:errorcluster, "UI ref."=w178:refnum<data-value>, "Data ref."=w179:refnum<data-value>, "Proceed?"=w182:bool)  [unwired: 5 in]
        n44 = Select(t=Main-actions."Acquire & process" ("MainStateSelector"), s=w182, f=Main-actions."Stop" ("MainStateSelector")) -> (s? t:f=w183:T30)
      }
      frame "Acquire & process" {
        # "Acquire, process, display and store images and data."
        n45 = call "Acquire-images.vi"("error in"=w196, "UI ref. in"=w198, "Data ref. in"=w197) -> ("error IO"=w189:errorcluster)  [unwired: 6 in, 2 out]
        n46 = call "Delay-processing.vi"("UI ref. in"=w198, "Data ref. in"=w197) -> ("error IO"=w190:errorcluster, "UI ref."=w193:refnum<data-value>, "Data ref."=w188:refnum<data-value>)  [unwired: 7 in]
        n47 = call "Update-and-display-processing-stats.vi"("Data ref. in"=w197, "UI ref. in"=w198) -> ("error IO"=w205:errorcluster)  [unwired: 7 in, 2 out]
        n48 = call "Update-and-display-module-status.vi"("Data ref. in"=w197, "UI ref. in"=w198) -> ("error IO"=w204:errorcluster)  [unwired: 7 in, 2 out]
        n49 = call "Update-main-display.vi"("Data ref. in"=w188, "UI ref. in"=w193) -> ("error IO"=w195:errorcluster)  [unwired: 7 in, 2 out]
        n50 = call "Update-characteristics-chart.vi"("Data ref. in"=w188, "UI ref. in"=w193) -> ("error IO"=w194:errorcluster)  [unwired: 7 in, 2 out]
        n51 = call "Process-images.vi"("UI ref. in"=w193, "Data ref. in"=w188) -> ("error IO"=w192:errorcluster)  [unwired: 7 in, 2 out]
        n52 = call "Filter-and-storage-wrapper.vi"("Data ref. in"=w188) -> ("error IO"=w191:errorcluster)  [unwired: 9 in, 1 out]
        n53 = call "Map-characteristics.vi"("Data ref. in"=w188) -> ("error out"=w187:errorcluster)  [unwired: 9 in, 1 out]
        n54 = Merge Errors(w192, w191, w187, w195, w194, w189, w190, w205, w204) -> (w202:errorcluster)
        n55 = call "Get-New-iteration.vi"("error in (no error)"=w202, "UI ref. in"=w198) -> ("error out"=w201:errorcluster, "New iteration"=w200:bool, "UI ref."=w199:refnum<data-value>)  [unwired: 7 in]
        n56 = Select(t=Main-actions."Iterate" ("MainStateSelector"), s=w200, f=Main-actions."Stop" ("MainStateSelector")) -> (s? t:f=w206:T30)
      }
      frame "Iterate" {
        w222 = FALSE  # Reset?
        # "Refresh the process and storage variables for a new acquisition iteration."
        n57 = call "Iterate-acquisition.vi"("error in"=w210, "Reset?"=w222, "Data ref. in"=w211) -> ("error IO"=w220:errorcluster, "Data ref."=w221:refnum<data-value>)  [unwired: 7 in]
        n58 = call "Update-processing-variables.vi"("error in (no error)"=w220, "Data ref. in"=w221) -> ("error out"=w216:errorcluster, "Data ref."=w215:refnum<data-value>)  [unwired: 8 in]
        n59 = call "Set-Iterate.vi"("error in (no error)"=w216, "Iterate"=FALSE, "UI ref. in"=w219) -> ("error out"=w212:errorcluster, "UI ref."=w213:refnum<data-value>)  [unwired: 7 in]
        n60 = call "Set-UI-state.vi"("State"=Application-states."Activated", "error in"=w212, "Data ref. in"=w215, "UI ref. in"=w213) -> ("error IO"=w217:errorcluster, "Data ref."=w214:refnum<data-value>, "UI ref."=w218:refnum<data-value>)  [unwired: 5 in]
      }
      frame "Stop" {
        w225 = FALSE  # Stop
        # "Release hardware resources and clear buffers where possible."
        n61 = call "Set-Acquisition.vi"("error in (no error)"=w227, "Acquisition"=w225, "UI ref. in"=w229) -> ("error out"=w226:errorcluster, "UI ref."=w228:refnum<data-value>)  [unwired: 7 in]
        n62 = call "Set-processing.vi"("error in (no error)"=w226, "Processing"=w225, "Data ref. in"=w241) -> ("error out"=w236:errorcluster, "Data ref."=w235:refnum<data-value>)  [unwired: 7 in]
        n63 = call "Release-hardware.vi"("error in (no error)"=w236, "Data ref. in"=w235) -> ("error out"=w233:errorcluster, "Data ref."=w234:refnum<data-value>)  [unwired: 8 in]
        n64 = call "Release-filter-file.vi"("error in"=w233, "Data ref. in"=w234) -> ("error IO"=w240:errorcluster, "Data ref."=w243:refnum<data-value>)  [unwired: 7 in, 1 out]
        n65 = call "Get-correlation-image-shift.vi"("error in"=w240, "Data ref. in"=w243) -> ("error IO"=w239:errorcluster, "Y-shift"=w244:i32, "X-shift"=w246:i32, "Data ref."=w242:refnum<data-value>)  [unwired: 6 in]
        n66 = call "Get-mapping-offset.vi"("error in"=w239, "Data ref. in"=w242) -> ("error IO"=w230:errorcluster, "Start offset"=w245:dbl, "Data ref."=w232:refnum<data-value>)  [unwired: 7 in]
        n67 = property on="X-shift" class="DigNum (strict)"("Value"=w246) -> ()  [unwired: 2 in, 2 out]
        n68 = property on="Y-shift" class="DigNum (strict)"("Value"=w244) -> ()  [unwired: 2 in, 2 out]
        n69 = property on="Start off-set" class="DigNum (strict)"("Value"=w245) -> ()  [unwired: 2 in, 2 out]
        n70 = call "Set-UI-state.vi"("State"=Application-states."Stopped", "error in"=w230, "Data ref. in"=w232, "UI ref. in"=w228) -> ("error IO"=w237:errorcluster, "Data ref."=w231:refnum<data-value>, "UI ref."=w238:refnum<data-value>)  [unwired: 5 in]
      }
      frame "Refresh display" {
        # "Refresh the display once, based on the current GUI selector values."
        # "Refresh the active display once, based on the display selector values."
        n71 = call "Update-main-display.vi"("error in"=w254, "Data ref. in"=w248, "UI ref. in"=w251) -> ("error IO"=w252:errorcluster, "Data ref."=w249:refnum<data-value>, "UI ref."=w250:refnum<data-value>)  [unwired: 6 in]
      }
      frame "Refresh status" {
        # "Refresh the module status once.."
        # "Refresh the module status overview once."
        n72 = call "Update-and-display-module-status.vi"("error in"=w255, "Data ref. in"=w259, "UI ref. in"=w260) -> ("error IO"=w256:errorcluster, "Data ref."=w258:refnum<data-value>, "UI ref."=w257:refnum<data-value>)  [unwired: 6 in]
      }
      frame "View camera settings" {
        # "Collect the settings of the currently selected camera and display in a (locking) dialog."
        n73 = call "View-camera-settings-with-dialog.vi"("error in (no error)"=w262, "UI ref. in"=w266, "Data ref. in"=w263) -> ("error out"=w264:errorcluster, "Data ref."=w265:refnum<data-value>)  [unwired: 7 in]
      }
      frame "View grabber settings" {
        # "Collect the settings of the framegrabber and display in a (locking) dialog."
        n74 = call "View-grabber-settings-with-dialog.vi"("error in (no error)"=w268, "UI ref. in"=w270, "Data ref. in"=w269) -> ("error out"=w271:errorcluster, "Data ref."=w272:refnum<data-value>)  [unwired: 7 in]
      }
      frame "Exit" {
        # "De-allocates the remaining memory buffers and checks the release of connected hardware."
        n75 = call "Set-Exit.vi"("error in (no error)"=w282, "Exit?"=TRUE, "UI ref. in"=w283) -> ("error out"=w275:errorcluster, "UI ref."=w278:refnum<data-value>)  [unwired: 7 in]
        n76 = call "Set-UI-state.vi"("State"=Application-states."Exited", "error in"=w275, "Data ref. in"=w279, "UI ref. in"=w278) -> ("error IO"=w276:errorcluster, "Data ref."=w280:refnum<data-value>, "UI ref."=w277:refnum<data-value>)  [unwired: 5 in]
      }
    }
    n77 = Format Into String(w31) -> (resulting string=→"Action":string)  [unwired: 3 in, 1 out]
    n78 = call "Get-exit.vi"("error in (no error)"=w36, "UI ref. in"=w35) -> ("error out"=w29:errorcluster, "Exit?"=w33:bool, "UI ref."=w30:refnum<data-value>)  [unwired: 7 in]
    n79 = Select(t=Main-actions."Exit", s=w33, f=w31) -> (s? t:f=w34:T30)
    n80 = call "Signal-error.vi"("error in (no error)"=w29, "Data ref. in"=w26) -> ("error out"=w28:errorcluster, "Data ref."=w27:refnum<data-value>)  [unwired: 8 in]
  }
  n81 = call "Register-events.vi"("error in (no error)"=w8, "Data ref. in"=w7) -> ("error out"=w9:errorcluster, "Events"=w4:refnum<event-registration>, "Data ref."=w10:refnum<data-value>)  [unwired: 7 in]
  n82 = while {
    shift-right: [w288] -> _
    shift-left: w15 -> [w297]
    shift-right: [w290] -> w12
    shift-left: w10 -> [w298]
    tunnel: w9 -> [w301]
    tunnel: [w291] -> w13
    shift-right: [w286] -> w3
    shift-left: w4 -> [w287]
    stop <- w294 stop-if-true
    # "User interface module"
    n83 = event shown="[18] Menu Selection (User)" {
      selector: w287 -> [_ _ _ _ _ _ _ _ _ _ _ _ _ _ _ _ _ _ _ _ _ _ _ _]
      dyn-events: [_ _ _ _ _ _ _ _ _ _ _ _ _ _ _ _ _ _ _ _ _ _ _ _] -> w286
      timeout: 1000 -> [_ _ _ _ _ _ _ _ _ _ _ _ _ _ _ _ _ _ _ _ _ _ _ _]
      tunnel: [_ _ _ _ _ _ _ _ _ _ _ _ _ _ _ _ _ _ _ _ TRUE ("notification") _ _ _] -> w300
      tunnel: [w302 w317 w319 w326 w334 w338 w350 w355 w357 w366 w371 w376 w384 w395 w402 w411 w415 w418 w429 w600 w606 w617 w620 w629] -> w296
      tunnel: w301 -> [w305 w318 w322 w329 w335 w342 w349 w354 w360 w367 w372 w380 w388 w396 w403 w412 w416 w421 w430 w601 w609 w617 w621 w630]
      tunnel: w298 -> [w306 w309 w323 w330 w336 w343 w346 w352 w361 w364 w373 w379 w389 w397 w404 w407 w413 w420 w428 w595 w610 w614 w622 w627]
      tunnel: w297 -> [w307 w308 w324 w331 w337 w344 w347 w353 w362 w365 w374 w382 w390 w398 w405 w408 w414 w423 w427 w596 w611 w615 w623 w628]
      tunnel: [w304 w308 w320 w328 w333 w340 w347 w353 w359 w365 w369 w378 w386 w394 w401 w410 w414 w419 w426 w596 w608 w615 w619 w626] -> w295
      tunnel: [w303 w310 w321 w327 w332 w339 w345 w351 w358 w363 w370 w377 w385 w393 w400 w409 w413 w420 w425 w595 w607 w614 w618 w625] -> w289
      event Timeout {
        # "Every second with no user action, the available disk space and moudle status is updated. The disk where the process information will be saved is used, rather than the disk where the program is located."
        n84 = event-data() -> ()  [unwired: 1 in, 3 out]
        n85 = call "Event-Timeout.vi"("error in (no error)"=w305, "Data ref. in"=w306, "UI ref. in"=w307) -> ("error out"=w302:errorcluster, "Data ref."=w303:refnum<data-value>, "UI ref."=w304:refnum<data-value>)  [unwired: 6 in]
      }
      event User Event {
        # "Every second with no user action, the available disk space and moudle status is updated. The disk where the process information will be saved is used, rather than the disk where the program is located."
        n86 = event-data() -> ("status"=w315:bool, "code"=w314:i32, "source"=w313:string)  [unwired: 1 in]
        n87 = Bundle By Name(cluster=errorcluster {"status"=FALSE, "code"=0, "source"=""} ("error constant"), "status"=w315, "code"=w314, "source"=w313) -> (w311:errorcluster)
        n88 = Merge Errors(w311, w318) -> (w312:errorcluster)
        n89 = call "Process-error.vi"("error in (no error)"=w312, "Data ref. in"=w309) -> ("error out"=w317:errorcluster, "Data ref."=w310:refnum<data-value>)  [unwired: 8 in]
      }
      event "Stop acquisition": Value Change {
        # "Signal the 'Acquisition' notifier with a 'stop' signal and set 'Stop' as the next program state if not in an active acquisition."
        n90 = event-data() -> ()  [unwired: 1 in, 1 out]
        n91 = call "Event-Stop.vi"("error in (no error)"=w322, "Data ref. in"=w323, "UI ref. in"=w324) -> ("error out"=w319:errorcluster, "Data ref."=w321:refnum<data-value>, "UI ref."=w320:refnum<data-value>)  [unwired: 6 in]
      }
      event "Displays": Value Change {
        # "Update the active display notifier to the display tab that the user selected (foreground tab).\nIf no acquisition is busy, force a display refresh."
        n92 = event-data() -> ("NewVal"=w325:T25)  [unwired: 1 in]
        n93 = call "Event-Display.vi"("Display"=w325, "error in (no error)"=w329, "Data ref. in"=w330, "UI ref. in"=w331) -> ("error out"=w326:errorcluster, "Data ref."=w327:refnum<data-value>, "UI ref."=w328:refnum<data-value>)  [unwired: 5 in]
      }
      event "Activate": Value Change {
        # "Prepare and activate the acquisition hardware. The current GUI settings will be checked, saved and locked."
        n94 = event-data() -> ()  [unwired: 1 in, 1 out]
        n95 = call "Event-Activate.vi"("error in (no error)"=w335, "Data ref. in"=w336, "UI ref. in"=w337) -> ("error out"=w334:errorcluster, "Data ref."=w332:refnum<data-value>, "UI ref."=w333:refnum<data-value>)  [unwired: 6 in]
      }
      event "Image refresh": Value Change {
        # "Signal the 'Image refresh' notifier. Check if an acquisition is busy. If no acquisition is ongoing, update the display. This will also reset the button to 'false', the refresh notifier will remain 'true'."
        n96 = event-data() -> ("NewVal"=w341:bool)  [unwired: 1 in]
        n97 = call "Event-Display-refresh.vi"("Display refresh"=w341, "error in (no error)"=w342, "Data ref. in"=w343, "UI ref. in"=w344) -> ("error out"=w338:errorcluster, "Data ref."=w339:refnum<data-value>, "UI ref."=w340:refnum<data-value>)  [unwired: 5 in]
      }
      event "Save settings": Value Change {
        w348 = T30[] [enum."Update settings", enum."Save settings with dialog"] items=["Idle", "Initialize", "Load defaults", "Update settings", "Check settings", "Save settings", "Save settings with dialog", "Load settings", "Load data", "Activate", "Start", "Wait for start signal", "Acquire & process", "Iterate", "Stop", "Refresh display", "Refresh status", "View camera settings", "View grabber settings", "Exit"] ("State array")
        # "Copy the GUI parameter values to the setting buffers, check the values for conflicts, save the values and return to the idle state."
        n98 = event-data() -> ()  [unwired: 1 in, 1 out]
        n99 = call "Enqueue-main-actions.vi"("error in (no error)"=w349, "State array"=w348, "Data ref. in"=w346) -> ("error out"=w350:errorcluster, "Data ref."=w345:refnum<data-value>)  [unwired: 6 in, 1 out]
      }
      event "Load settings": Value Change {
        w356 = T30[] [enum."Load settings"] items=["Idle", "Initialize", "Load defaults", "Update settings", "Check settings", "Save settings", "Save settings with dialog", "Load settings", "Load data", "Activate", "Start", "Wait for start signal", "Acquire & process", "Iterate", "Stop", "Refresh display", "Refresh status", "View camera settings", "View grabber settings", "Exit"] ("State array")
        # "Set the 'Load settings' program state chain. The settings are first loaded, according to the 'Settings source' value, the settings are then copied from the GUI to the buffer and the settings are checked for consistency."
        n100 = event-data() -> ()  [unwired: 1 in, 1 out]
        n101 = call "Enqueue-main-actions.vi"("error in (no error)"=w354, "State array"=w356, "Data ref. in"=w352) -> ("error out"=w355:errorcluster, "Data ref."=w351:refnum<data-value>)  [unwired: 6 in, 1 out]
      }
      event "Start acquisition": Value Change {
        # "Starts the hardware acquisition. The actual start may be delayed, based on the 'acquisition' settings."
        n102 = event-data() -> ()  [unwired: 1 in, 1 out]
        n103 = call "Event-Start.vi"("error in (no error)"=w360, "Data ref. in"=w361, "UI ref. in"=w362) -> ("error out"=w357:errorcluster, "Data ref."=w358:refnum<data-value>, "UI ref."=w359:refnum<data-value>)  [unwired: 6 in]
      }
      event "Import images": Value Change {
        w368 = T30[] [enum."Load data"] items=["Idle", "Initialize", "Load defaults", "Update settings", "Check settings", "Save settings", "Save settings with dialog", "Load settings", "Load data", "Activate", "Start", "Wait for start signal", "Acquire & process", "Iterate", "Stop", "Refresh display", "Refresh status", "View camera settings", "View grabber settings", "Exit"]
        # "Set the next program state to 'Import data' to import images or remove previously imported images. Importing images will set the acquisition state to 'simulation'."
        n104 = event-data() -> ()  [unwired: 1 in, 1 out]
        n105 = call "Enqueue-main-actions.vi"("error in (no error)"=w367, "State array"=w368, "Data ref. in"=w364) -> ("error out"=w366:errorcluster, "Data ref."=w363:refnum<data-value>)  [unwired: 6 in, 1 out]
      }
      event "Batch browser": Value Change {
        # "Signal the newly chosen batch image to the 'Timestep' notifier. Refresh the display when no acquisition is ongoing."
        n106 = event-data() -> ("NewVal"=w375:i32)  [unwired: 1 in]
        n107 = call "Event-Timestep.vi"("Timestep"=w375, "error in (no error)"=w372, "Data ref. in"=w373, "UI ref. in"=w374) -> ("error out"=w371:errorcluster, "Data ref."=w370:refnum<data-value>, "UI ref."=w369:refnum<data-value>)  [unwired: 5 in]
      }
      event Value Change {
        # "Update the enabled state of the 'Load settings' button when the user changes the 'Settings source' control value. Also update the new settings source value to its notifier."
        n108 = event-data() -> ("NewVal"=w381:T3)  [unwired: 1 in]
        n109 = call "Event-Settings-source.vi"("Settings source"=w381, "error in (no error)"=w380, "Data ref. in"=w379, "UI ref. in"=w382) -> ("error out"=w376:errorcluster, "Data ref."=w377:refnum<data-value>, "UI ref."=w378:refnum<data-value>)  [unwired: 5 in]
      }
      event Value Change {
        # "Update the display image type notifier to the user selected value.\nIf no acquisition is busy, force a display refresh."
        n110 = event-data() -> ("NewVal"=w387:T2)  [unwired: 1 in]
        n111 = Current VI's Menubar() -> (w383:refnum<k9>)
        n112 = call "Event-Image-type.vi"("Menu ref."=w383, "Image type"=w387, "error in (no error)"=w388, "Data ref. in"=w389, "UI ref. in"=w390) -> ("error out"=w384:errorcluster, "Data ref."=w385:refnum<data-value>, "UI ref."=w386:refnum<data-value>)  [unwired: 4 in]
      }
      event Value Change {
        # "Update the camera index notifier to the user selected value.\nIf no acquisition is busy, force a display refresh."
        n113 = event-data() -> ("NewVal"=w392:T1)  [unwired: 1 in]
        n114 = Current VI's Menubar() -> (w391:refnum<k9>)
        n115 = call "Event-Camera.vi"("Menu ref."=w391, "Camera"=w392, "error in (no error)"=w396, "Data ref. in"=w397, "UI ref. in"=w398) -> ("error out"=w395:errorcluster, "Data ref."=w393:refnum<data-value>, "UI ref."=w394:refnum<data-value>)  [unwired: 4 in]
      }
      event Value Change {
        # "Enable or disable and reset the 'Camera selector' button based on the new value of the 'Number of cameras' control."
        n116 = event-data() -> ("NewVal"=w399:i32)  [unwired: 1 in]
        n117 = call "Event-Camera-amount.vi"("# cameras"=w399, "error in (no error)"=w403, "Data ref. in"=w404, "UI ref. in"=w405) -> ("error out"=w402:errorcluster, "Data ref."=w400:refnum<data-value>, "UI ref."=w401:refnum<data-value>)  [unwired: 5 in]
      }
      event Value Change {
        # "Update the enabled state of the 'Browse batch' control when the user changes the value of the 'Acquisition mode' GUI control."
        n118 = event-data() -> ("NewVal"=w406:T32)  [unwired: 1 in]
        n119 = call "Event-Acquisition-mode.vi"("Acquis. mode"=w406, "error in (no error)"=w412, "Data ref. in"=w407, "UI ref. in"=w408) -> ("error out"=w411:errorcluster, "Data ref."=w409:refnum<data-value>, "UI ref."=w410:refnum<data-value>)  [unwired: 5 in]
      }
      event "Processing selector": Value Change {
        # "Change the visible parameter group on the 'Processing' tab."
        n120 = event-data() -> ("NewVal"=w417:u32)  [unwired: 1 in]
        n121 = property on="Processing tabs" class="TabCtl (strict)"(error in=w416, "Value"=w417) -> (error out=w415:errorcluster)  [unwired: 1 in, 1 out]
      }
      event Value Change {
        # "Update the 'Map characteristic' notifier to the new, user selected value."
        n122 = event-data() -> ("NewVal"=w422:T16)  [unwired: 1 in]
        n123 = call "Set-Map-characteristic-notif.vi"("error in (no error)"=w421, "Map characteristic"=w422, "UI ref. in"=w423) -> ("error out"=w418:errorcluster, "UI ref."=w419:refnum<data-value>)  [unwired: 7 in]
      }
      event Menu Selection (User) {
        # "Perform the actions associated to the user menu event."
        n124 = event-data() -> ("MenuRef"=w424:refnum<k9>, "ItemTag"=w431:string)  [unwired: 1 in]
        n125 = case shown="\"CV_ACTIVATE\"" w431 {
          selector: w431 -> [_ _ _ _ _ _ _ _ _ _ _ _ _ w533 w538 _ _ _ _ _ _ _ _ _]
          tunnel: w430 -> [w436 w443 w449 w457 w467 w477 w483 w487 w495 w496 w509 w515 w523 w530 w541 w544 w547 w552 w560 w568 w576 w582 w586 w592]
          tunnel: [w435 w441 w452 w456 w465 w473 w480 w486 w490 w497 w502 w514 w522 w529 w535 w544 w547 w551 w559 w565 w575 w582 w585 w591] -> w429
          tunnel: w428 -> [w433 w439 w445 w454 w463 w471 w482 w488 w494 w501 w507 w516 w524 w531 w540 w542 w545 w553 w561 w569 w577 w580 w587 w593]
          tunnel: w427 -> [w434 w440 w447 w458 w466 w472 w481 w489 w493 w500 w508 w517 w525 w532 w539 w543 w546 w554 w562 w570 w578 w581 w588 w594]
          tunnel: [w434 w440 w446 w455 w464 w472 w479 w485 w492 w499 w506 w513 w521 w527 w537 w543 w546 w550 w558 w567 w573 w581 w583 w589] -> w426
          tunnel: [w432 w438 w444 w453 w462 w471 w478 w484 w491 w498 w505 w512 w520 w528 w536 w542 w545 w549 w557 w566 w574 w580 w584 w590] -> w425
          tunnel: w424 -> [_ _ _ _ _ _ _ _ _ _ _ _ w518 w526 w534 _ _ w548 w556 w564 w572 _ _ _]
          frame "CV_SAVE" {
            w437 = T30[] [enum."Update settings", enum."Save settings"] items=["Idle", "Initialize", "Load defaults", "Update settings", "Check settings", "Save settings", "Save settings with dialog", "Load settings", "Load data", "Activate", "Start", "Wait for start signal", "Acquire & process", "Iterate", "Stop", "Refresh display", "Refresh status", "View camera settings", "View grabber settings", "Exit"]
            n126 = call "Enqueue-main-actions.vi"("error in (no error)"=w436, "State array"=w437, "Data ref. in"=w433) -> ("error out"=w435:errorcluster, "Data ref."=w432:refnum<data-value>)  [unwired: 6 in, 1 out]
          }
          frame "CV_CHECK_SETTINGS" {
            w442 = T30[] [enum."Update settings"] items=["Idle", "Initialize", "Load defaults", "Update settings", "Check settings", "Save settings", "Save settings with dialog", "Load settings", "Load data", "Activate", "Start", "Wait for start signal", "Acquire & process", "Iterate", "Stop", "Refresh display", "Refresh status", "View camera settings", "View grabber settings", "Exit"]
            n127 = call "Enqueue-main-actions.vi"("error in (no error)"=w443, "State array"=w442, "Data ref. in"=w439) -> ("error out"=w441:errorcluster, "Data ref."=w438:refnum<data-value>)  [unwired: 6 in, 1 out]
          }
          frame "CV_LOAD_DEFAULTS" {
            w448 = Settings-source."Default"  # Settings source
            w451 = T30[] [enum."Load settings"] items=["Idle", "Initialize", "Load defaults", "Update settings", "Check settings", "Save settings", "Save settings with dialog", "Load settings", "Load data", "Activate", "Start", "Wait for start signal", "Acquire & process", "Iterate", "Stop", "Refresh display", "Refresh status", "View camera settings", "View grabber settings", "Exit"]
            n128 = call "Set-Settings-notif.vi"("error in (no error)"=w449, "Settings source"=w448, "UI ref. in"=w447) -> ("error out"=w450:errorcluster, "UI ref."=w446:refnum<data-value>)  [unwired: 7 in]
            n129 = call "Enqueue-main-actions.vi"("error in (no error)"=w450, "State array"=w451, "Data ref. in"=w445) -> ("error out"=w452:errorcluster, "Data ref."=w444:refnum<data-value>)  [unwired: 6 in, 1 out]
          }
          frame "CV_LOAD_LAST" {
            w459 = Settings-source."Last used"  # Settings source
            w461 = T30[] [enum."Load settings"] items=["Idle", "Initialize", "Load defaults", "Update settings", "Check settings", "Save settings", "Save settings with dialog", "Load settings", "Load data", "Activate", "Start", "Wait for start signal", "Acquire & process", "Iterate", "Stop", "Refresh display", "Refresh status", "View camera settings", "View grabber settings", "Exit"]
            n130 = call "Set-Settings-notif.vi"("error in (no error)"=w457, "Settings source"=w459, "UI ref. in"=w458) -> ("error out"=w460:errorcluster, "UI ref."=w455:refnum<data-value>)  [unwired: 7 in]
            n131 = call "Enqueue-main-actions.vi"("error in (no error)"=w460, "State array"=w461, "Data ref. in"=w454) -> ("error out"=w456:errorcluster, "Data ref."=w453:refnum<data-value>)  [unwired: 6 in, 1 out]
          }
          frame "CV_LOAD_FILE" {
            w468 = Settings-source."File"  # Settings source
            w470 = T30[] [enum."Load settings"] items=["Idle", "Initialize", "Load defaults", "Update settings", "Check settings", "Save settings", "Save settings with dialog", "Load settings", "Load data", "Activate", "Start", "Wait for start signal", "Acquire & process", "Iterate", "Stop", "Refresh display", "Refresh status", "View camera settings", "View grabber settings", "Exit"]
            n132 = call "Set-Settings-notif.vi"("error in (no error)"=w467, "Settings source"=w468, "UI ref. in"=w466) -> ("error out"=w469:errorcluster, "UI ref."=w464:refnum<data-value>)  [unwired: 7 in]
            n133 = call "Enqueue-main-actions.vi"("error in (no error)"=w469, "State array"=w470, "Data ref. in"=w463) -> ("error out"=w465:errorcluster, "Data ref."=w462:refnum<data-value>)  [unwired: 6 in, 1 out]
          }
          frame "CV_IMPORT" {
            n134 = property on="Import images" class="Bool (strict)"(error in=w477) -> (error out=w476:errorcluster, "Value"=w475:bool)  [unwired: 1 in, 1 out]
            n135 = Not(x=w475) -> (.not. x?=w474:bool)
            n136 = property on="Import images" class="Bool (strict)"(error in=w476, "Val(Sgnl)"=w474) -> (error out=w473:errorcluster)  [unwired: 1 in, 1 out]
          }
          frame "CV_START" {
            n137 = call "Event-Start.vi"("error in (no error)"=w483, "Data ref. in"=w482, "UI ref. in"=w481) -> ("error out"=w480:errorcluster, "Data ref."=w478:refnum<data-value>, "UI ref."=w479:refnum<data-value>)  [unwired: 6 in]
          }
          frame "CV_ITERATE" {
            n138 = call "Event-Iterate.vi"("error in (no error)"=w487, "Data ref. in"=w488, "UI ref. in"=w489) -> ("error out"=w486:errorcluster, "Data ref."=w484:refnum<data-value>, "UI ref."=w485:refnum<data-value>)  [unwired: 6 in]
          }
          frame "CV_STOP" {
            n139 = call "Event-Stop.vi"("error in (no error)"=w495, "Data ref. in"=w494, "UI ref. in"=w493) -> ("error out"=w490:errorcluster, "Data ref."=w491:refnum<data-value>, "UI ref."=w492:refnum<data-value>)  [unwired: 6 in]
          }
          frame "CV_ACTIVATE" {
            n140 = call "Event-Activate.vi"("error in (no error)"=w496, "Data ref. in"=w501, "UI ref. in"=w500) -> ("error out"=w497:errorcluster, "Data ref."=w498:refnum<data-value>, "UI ref."=w499:refnum<data-value>)  [unwired: 6 in]
          }
          frame "CV_REFRESH" {
            n141 = property on="Image refresh" class="Bool (strict)"(error in=w509) -> (error out=w510:errorcluster, "Value"=w511:bool)  [unwired: 1 in, 1 out]
            n142 = Not(x=w511) -> (.not. x?=w504:bool)
            n143 = call "Event-Display-refresh.vi"("Display refresh"=w504, "error in (no error)"=w510, "Data ref. in"=w507, "UI ref. in"=w508) -> ("error out"=w503:errorcluster, "Data ref."=w505:refnum<data-value>, "UI ref."=w506:refnum<data-value>)  [unwired: 5 in]
            n144 = property on="Image refresh" class="Bool (strict)"(error in=w503, "Value"=w504) -> (error out=w502:errorcluster)  [unwired: 1 in, 1 out]
          }
          frame "CV_SNAPSHOT" {
            n145 = call "Event-Snapshot.vi"("error in (no error)"=w515, "Data ref. in"=w516, "UI ref. in"=w517) -> ("error out"=w514:errorcluster, "Data ref."=w512:refnum<data-value>, "UI ref."=w513:refnum<data-value>)  [unwired: 6 in]
          }
          frame "CV_CAM2" {
            w519 = Camera-selector."Camera 2"  # Camera
            n146 = call "Event-Camera.vi"("Menu ref."=w518, "Camera"=w519, "error in (no error)"=w523, "Data ref. in"=w524, "UI ref. in"=w525) -> ("error out"=w522:errorcluster, "Data ref."=w520:refnum<data-value>, "UI ref."=w521:refnum<data-value>)  [unwired: 4 in]
          }
          frame "CV_TOOLBAR" {
            n147 = call "Event-Toolbar.vi"("Menu ref."=w526, "Tag"=w533, "error in (no error)"=w530, "Data ref. in"=w531, "UI ref. in"=w532) -> ("error out"=w529:errorcluster, "Data ref."=w528:refnum<data-value>, "UI ref."=w527:refnum<data-value>)  [unwired: 4 in]
          }
          frame "CV_SETTINGS" {
            n148 = call "Event-Settings-bar.vi"("Menu ref."=w534, "Tag"=w538, "error in (no error)"=w541, "Data ref. in"=w540, "UI ref. in"=w539) -> ("error out"=w535:errorcluster, "Data ref."=w536:refnum<data-value>, "UI ref."=w537:refnum<data-value>)  [unwired: 4 in]
          }
          frame "CV_UI_DEFAULTS" {
            n149 = call "Edit-GUI-param-defaults-with-dialog.vi"() -> ()  [unwired: 12 in]
          }
          frame "CV_ADVANCED_DEFAULTS" {
            n150 = call "Edit-advanced-param-defaults-with-dialog.vi"() -> ()  [unwired: 12 in]
          }
          frame "CV_CAM1" {
            w555 = Camera-selector."Camera 1"  # Camera
            n151 = call "Event-Camera.vi"("Menu ref."=w548, "Camera"=w555, "error in (no error)"=w552, "Data ref. in"=w553, "UI ref. in"=w554) -> ("error out"=w551:errorcluster, "Data ref."=w549:refnum<data-value>, "UI ref."=w550:refnum<data-value>)  [unwired: 4 in]
          }
          frame "CV_ORIGINAL" {
            n152 = call "Event-Image-type.vi"("Menu ref."=w556, "Image type"=Image-selector."Original" ("Value (Signaling)"), "error in (no error)"=w560, "Data ref. in"=w561, "UI ref. in"=w562) -> ("error out"=w559:errorcluster, "Data ref."=w557:refnum<data-value>, "UI ref."=w558:refnum<data-value>)  [unwired: 4 in]
          }
          frame "CV_CORRECTED" {
            n153 = call "Event-Image-type.vi"("Menu ref."=w564, "Image type"=Image-selector."Corrected" ("Value (Signaling)"), "error in (no error)"=w568, "Data ref. in"=w569, "UI ref. in"=w570) -> ("error out"=w565:errorcluster, "Data ref."=w566:refnum<data-value>, "UI ref."=w567:refnum<data-value>)  [unwired: 4 in]
          }
          frame "CV_BINARY" {
            n154 = call "Event-Image-type.vi"("Menu ref."=w572, "Image type"=Image-selector."Binary" ("Value (Signaling)"), "error in (no error)"=w576, "Data ref. in"=w577, "UI ref. in"=w578) -> ("error out"=w575:errorcluster, "Data ref."=w574:refnum<data-value>, "UI ref."=w573:refnum<data-value>)  [unwired: 4 in]
          }
          frame Default {
          }
          frame "CV_CAMERA_SETTINGS" {
            n155 = call "Event-View-camera-settings.vi"("error in (no error)"=w586, "Data ref. in"=w587, "UI ref. in"=w588) -> ("error out"=w585:errorcluster, "Data ref."=w584:refnum<data-value>, "UI ref."=w583:refnum<data-value>)  [unwired: 6 in]
          }
          frame "CV_GRABBER_SETTINGS" {
            n156 = call "Event-View-grabber-settings.vi"("error in (no error)"=w592, "Data ref. in"=w593, "UI ref. in"=w594) -> ("error out"=w591:errorcluster, "Data ref."=w590:refnum<data-value>, "UI ref."=w589:refnum<data-value>)  [unwired: 6 in]
          }
        }
      }
      event Mouse Down? {
        # "Reset the GUI controls for the image size (ROI) to the maximum image size."
        n157 = event-data() -> ()  [unwired: 1 in, 3 out]
        n158 = control-ref of="ROI width"() -> (w597:refnum<vi>)
        n159 = control-ref of="ROI height"() -> (w598:refnum<vi>)
        n160 = property class="DigNum (strict)"(reference=w597, error in=w601, "Val(Sgnl)"=u32 1248 ("Value")) -> (error out=w599:errorcluster)  [unwired: 1 out]
        n161 = property class="DigNum (strict)"(reference=w598, error in=w601, "Val(Sgnl)"=u32 1082 ("Value (Signaling)")) -> (error out=w605:errorcluster)  [unwired: 1 out]
        n162 = event-data("Discard?"=TRUE) -> ()  [unwired: 1 in, 1 out]
        n163 = Merge Errors(w599, w605) -> (w600:errorcluster)
      }
      event Panel Close? {
        # "The user wants to shut down the program. Intercept the normal shutdown and set 'Exit' as the next program state. Delete any waiting program states. Signal the 'Stop' notifier to abort an ongoing acquisition. End the user interface module to ignore any new input."
        n164 = event-data() -> ()  [unwired: 1 in, 1 out]
        n165 = call "Event-Exit.vi"("error in (no error)"=w609, "Data ref. in"=w610, "UI ref. in"=w611) -> ("error out"=w606:errorcluster, "Data ref."=w607:refnum<data-value>, "UI ref."=w608:refnum<data-value>)  [unwired: 6 in]
        n166 = event-data("Discard?"=TRUE) -> ()  [unwired: 1 in, 1 out]
      }
      event "Show info": Value Change {
        # "Show or hide the context help window."
        n167 = event-data() -> ("NewVal"=w616:bool)  [unwired: 1 in]
        n168 = Control Help Window(1:w616) -> ()  [unwired: 1 in]
      }
      event Value Change {
        # "Update the enabled state of the 'Manual trigger' button when the user changes the value of the 'Trigger mode'. The button is only enabled when the triggering is manual."
        n169 = event-data() -> ("NewVal"=w624:T7)  [unwired: 1 in]
        n170 = call "Event-Trigger-mode.vi"("Trigger mode"=w624, "error in (no error)"=w621, "Data ref. in"=w622, "UI ref. in"=w623) -> ("error out"=w620:errorcluster, "Data ref."=w618:refnum<data-value>, "UI ref."=w619:refnum<data-value>)  [unwired: 5 in]
      }
      event "Manual trigger": Value Change {
        # "Sends a trigger signal to the acquisition timed loop, if 'manual' triggering is selected as the acquisition mode and an acquisition is active."
        n171 = event-data() -> ()  [unwired: 1 in, 1 out]
        n172 = call "Event-Snapshot.vi"("error in (no error)"=w630, "Data ref. in"=w627, "UI ref. in"=w628) -> ("error out"=w629:errorcluster, "Data ref."=w625:refnum<data-value>, "UI ref."=w626:refnum<data-value>)  [unwired: 6 in]
      }
    }
    n173 = call "Get-exit.vi"("error in (no error)"=w296, "UI ref. in"=w295) -> ("error out"=w292:errorcluster, "Exit?"=w293:bool, "UI ref."=w288:refnum<data-value>)  [unwired: 7 in]
    n174 = Or(x=w300, y=w293) -> (x .or. y?=w294:bool)
    n175 = call "Signal-error.vi"("error in (no error)"=w292, "Data ref. in"=w289) -> ("error out"=w291:errorcluster, "Data ref."=w290:refnum<data-value>)  [unwired: 8 in]
  }
  n176 = call "Message-handler.vi"("error in (no error)"=w8, "UI ref. in"=w15, "Data ref. in"=w7) -> ("error out"=w16:errorcluster)  [unwired: 6 in, 2 out]
  n177 = call "Unregister-events.vi"("error in (no error)"=w13, "Events"=w3, "Data ref. in"=w12) -> ("error out"=w11:errorcluster)  [unwired: 7 in, 1 out]
  n178 = Merge Errors(w16, w11, w18) -> (w17:errorcluster)
  n179 = call "Clear-object.vi"("error in"=w17, "UI ref."=w20) -> ("error IO"=w19:errorcluster)  [unwired: 9 in]
  n180 = call "Clear-object.vi"("error in (no error)"=w19, "Data ref."=w22) -> ("error out"=w6:errorcluster)  [unwired: 9 in]
  n181 = call "Close-GUI.vi"("error in (no error)"=w6) -> ("error out"=→"error out":errorcluster)  [unwired: 10 in]
